vi "Initialise IO.vi"(8 "error in (no error)":errorcluster) -> (0 "error out":errorcluster, 3 "IO":T1)   [LabVIEW 2021]
uses:
  IO_Type.ctl
  <vilib>/TSA/Event Log/Event_TextLog/Event_TextLog.lvclass
  Blackboard/Blackboard.lvclass
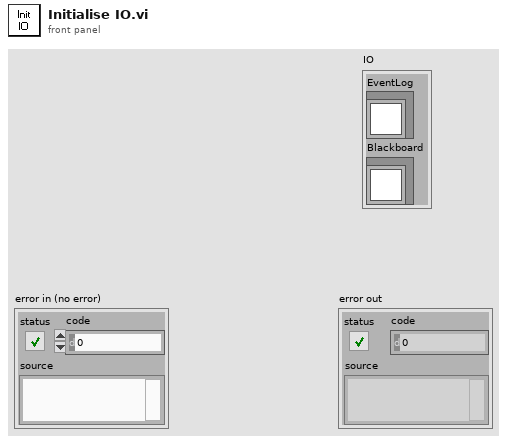
[diagram p1: front panel]
types:
  T1 = typedef "IO_Type.ctl" = cluster{"EventLog":refnum<class "Event_TextLog.lvclass">, "Blackboard":refnum<class "Blackboard.lvclass">}
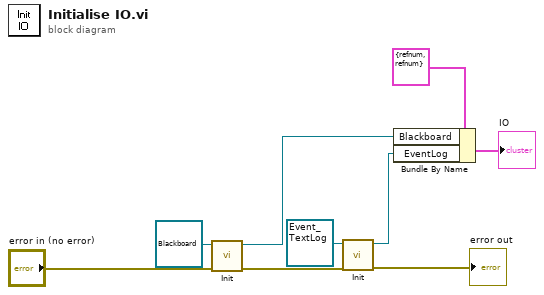
[diagram p0: block diagram]
diagram:
  n1 = call-dynamic "Init.vi"("error in (no error)"="error in (no error)", "bt_Blackboard in"=refnum<class "Blackboard.lvclass"> refnum) -> ("error out"=w3:errorcluster, "bt_Blackboard out"=w2:refnum<class "Blackboard.lvclass">)  [unwired: 8 in]
  n2 = call-dynamic "Init.vi"("error in (no error)"=w3, "Event_TextLog in"=refnum<class "Event_TextLog.lvclass"> refnum) -> ("error out"=→"error out":errorcluster, "Event_TextLog out"=w5:refnum<class "Event_TextLog.lvclass">)  [unwired: 8 in]
  n3 = Bundle By Name(cluster=T1 {"EventLog"=refnum, "Blackboard"=refnum} ("IO"), "Blackboard"=w2, "EventLog"=w5) -> (→"IO":T1)
